vi "make_path_relative.vi"(8 "error in (no error)":errorcluster, 10 "base":path, 11 "folder in":path) -> (0 "error out":errorcluster, 3 "folder out":path)   [LabVIEW 2015]
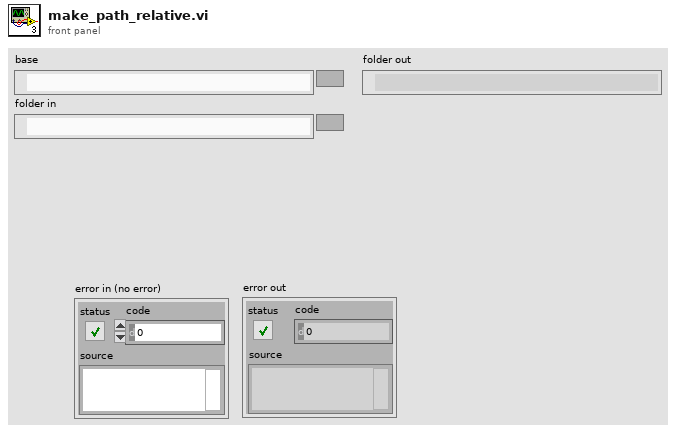
[diagram p1: front panel]
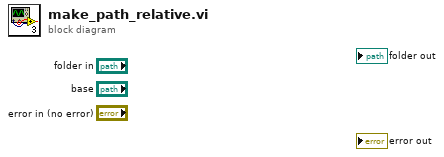
[diagram p0: block diagram]
diagram:
